vi "get Control State.vi"(11 "Ship in":refnum<class "Ship.lvclass">) -> (3 "Control State":refnum<class "Control State.lvclass">)   [LabVIEW 2021, in "Ship.lvclass"]
uses:
  Ship.lvclass
  Control State/Control State.lvclass
  Ship.lvclass/Ship.ctl
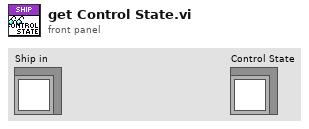
[diagram p1: front panel]
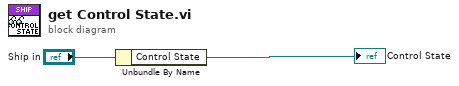
[diagram p0: block diagram]
diagram:
  n1 = Unbundle By Name("Ship in") -> ("Control State"=→"Control State":refnum<class "Control State.lvclass">)
